vi "Queue Driver.vi"(0 "States[]":string[](array[string]), 11 "Error In":errorcluster, 13 "Operation":T1) -> (4 "Dequeue Element":string, 15 "Error Out":errorcluster)   [LabVIEW 2019]
doc: "The VI performs the queue operations. The operations include create, enqueue, dequeue, enstack. flush and releases the queue."
uses:
  Typedef/Queue Operation.ctl
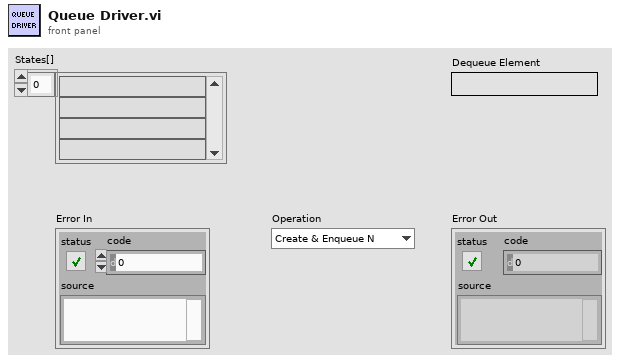
[diagram p1: front panel]
types:
  T1 = typedef "Queue Operation.ctl" = enum16{"Create & Enqueue N", "Enqueue N", "Dequeue", "Enstack N", "Flush", "Release"}
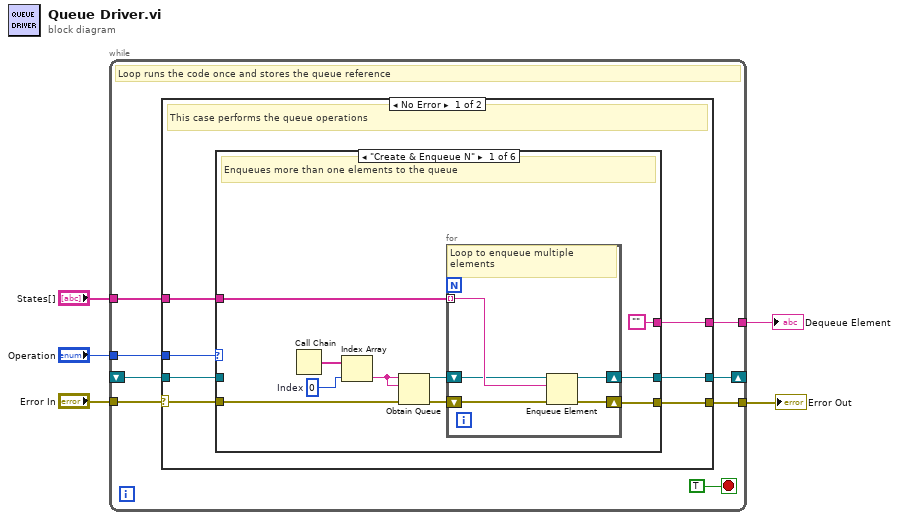
[diagram p0: block diagram]
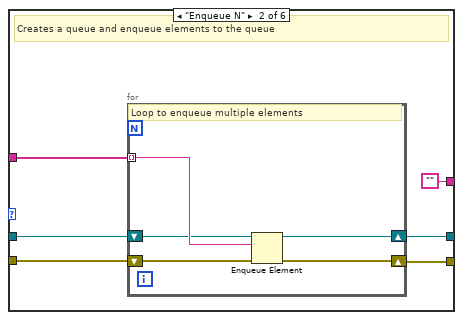
[diagram p2: hidden frame]
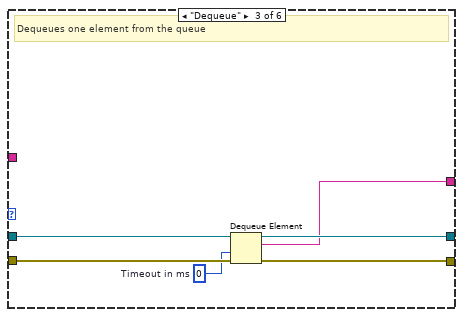
[diagram p3: hidden frame]
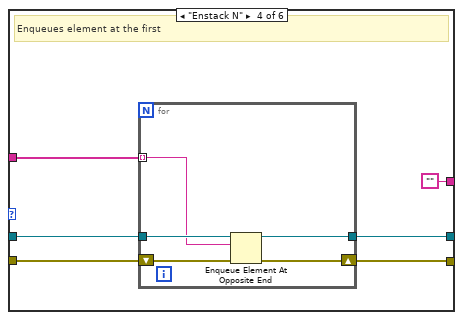
[diagram p4: hidden frame]
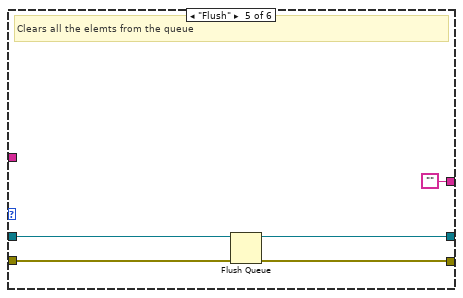
[diagram p5: hidden frame]
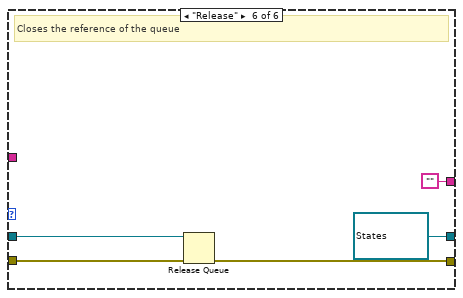
[diagram p6: hidden frame]
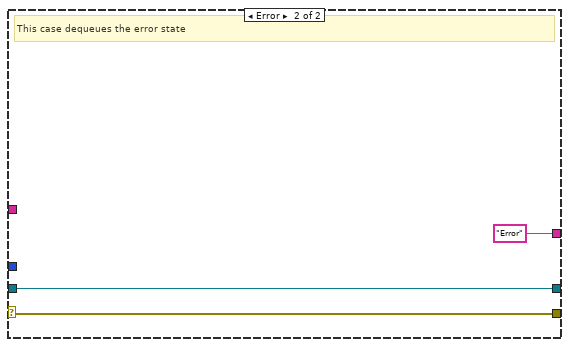
[diagram p7: hidden frame]
diagram:
  n1 = while {
    tunnel: "Error In" -> [w13]
    tunnel: "Operation" -> [w12]
    tunnel: "States[]" -> [w11]
    shift-right: [w10] -> _
    shift-left: _ -> [w9]
    tunnel: [w8] -> w2
    tunnel: [w6] -> w1
    stop <- TRUE stop-if-true
    # "Loop runs the code once and stores the queue reference"
    n2 = case shown="No Error" w13 {
      selector: w13 -> [w20 w75]
      tunnel: w12 -> [w19 _]
      tunnel: w11 -> [w18 _]
      tunnel: [w17 w76] -> w10
      tunnel: w9 -> [w16 w76]
      tunnel: [w15 w75] -> w8
      tunnel: [w14 "Error" ("Queue Name")] -> w6
      frame No Error {
        # "This case performs the queue operations"
        n3 = case shown="\"Create & Enqueue N\"" w19 {
          tunnel: [w30 w40 w51 w57 w67 w72] -> w15
          tunnel: w20 -> [w23 w41 w52 w58 w68 w73]
          tunnel: w18 -> [w29 w39 _ w53 _ _]
          tunnel: [w28 w37 w50 w55 w65 refnum<queue> refnum ("queue out")] -> w17
          tunnel: w16 -> [_ w38 w49 w56 w66 w71]
          tunnel: ["" ("States") "" ("States") w47 "" ("States") "" ("States") "" ("States")] -> w14
          frame "Create & Enqueue N" {
            w24 = 0  # Index
            # "Enqueues more than one elements to the queue"
            n4 = Call Chain() -> (call chain=w25:string[])
            n5 = Index Array(array=w25, index=w24) -> (element=w26:string)
            n6 = Obtain Queue(name (unnamed)=w26, element data type=w26, error in (no error)=w23) -> (queue out=w21:refnum<queue>, error out=w22:errorcluster)  [unwired: 2 in, 1 out]
            n7 = for {
              shift-right: [w34] -> w30
              shift-left: w22 -> [w35]
              tunnel: w29 -> [w33] mode=indexing
              shift-right: [w31] -> w28
              shift-left: w21 -> [w32]
              # "Loop to enqueue multiple elements"
              n8 = Enqueue Element(queue=w32, element=w33, error in (no error)=w35) -> (queue out=w31:refnum<queue>, error out=w34:errorcluster)  [unwired: 1 in, 1 out]
            }
          }
          frame "Enqueue N" {
            # "Creates a queue and enqueue elements to the queue"
            n9 = for {
              shift-right: [w45] -> w40
              shift-left: w41 -> [w46]
              tunnel: w39 -> [w44] mode=indexing
              shift-right: [w42] -> w37
              shift-left: w38 -> [w43]
              # "Loop to enqueue multiple elements"
              n10 = Enqueue Element(queue=w43, element=w44, error in (no error)=w46) -> (queue out=w42:refnum<queue>, error out=w45:errorcluster)  [unwired: 1 in, 1 out]
            }
          }
          frame "Dequeue" {
            w48 = 0  # Timeout in ms
            # "Dequeues one element from the queue"
            n11 = Dequeue Element(queue=w49, timeout in ms (-1)=w48, error in (no error)=w52) -> (queue out=w50:refnum<queue>, element=w47:string, error out=w51:errorcluster)  [unwired: 1 out]
          }
          frame "Enstack N" {
            # "Enqueues element at the first"
            n12 = for {
              tunnel: w56 -> [w61]
              tunnel: [w60] -> w55
              shift-right: [w62] -> w57
              shift-left: w58 -> [w63]
              tunnel: w53 -> [w59] mode=indexing
              n13 = Enqueue Element At Opposite End(queue=w61, element=w59, error in (no error)=w63) -> (queue out=w60:refnum<queue>, error out=w62:errorcluster)  [unwired: 1 in, 1 out]
            }
          }
          frame "Flush" {
            # "Clears all the elemts from the queue"
            n14 = Flush Queue(queue=w66, error in (no error)=w68) -> (queue out=w65:refnum<queue>, error out=w67:errorcluster)  [unwired: 1 out]
          }
          frame "Release" {
            # "Closes the reference of the queue"
            n15 = Release Queue(queue=w71, error in (no error)=w73) -> (error out=w72:errorcluster)  [unwired: 1 in, 2 out]
          }
        }
      }
      frame Error {
        # "This case dequeues the error state"
      }
    }
  }
  "Error Out" <- w2
  "Dequeue Element" <- w1
